vi "Set Voltage and Current.vi"(0 "reference in":refnum<class "Power Supply.lvclass">, 3 "Set Voltage (V)":dbl=5.0, 4 "Set Current (A)":dbl=1.0, 5 "error in (no error)":errorcluster) -> (14 "reference out":refnum<class "Power Supply.lvclass">, 19 "error out":errorcluster)   [LabVIEW 2017, in "Power Supply.lvclass"]
uses:
  Power Supply.lvclass
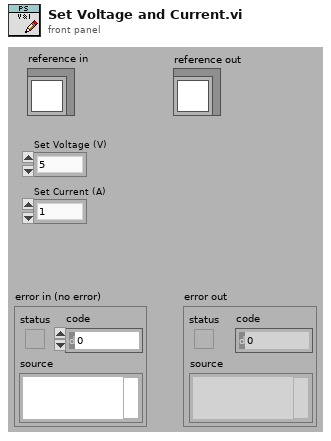
[diagram p1: front panel]
types:
  T1 = typedef "Power Supply.lvclass/ObjectAttributes.ctl" = cluster{"Power Supply Chain VISA Session":refnum<visa-resource-name>, "Power Supply Chain Address":i16, "Power Supply Open/Close Status":bool, "Power Supply Voltage Setting":dbl, "Power Supply Current Setting":dbl, "Power Supply Voltage Reading":dbl, "Power Supply Current Reading":dbl, "Power Supply Status":T2, "Power Supply Error":T3, "Fault Register":u8, "Power Supply Error":bool}
  T2 = typedef "Power Supply.lvclass/Power Supply Status.ctl" = enum16{"Closed", "Open"}
  T3 = typedef "Power Supply.lvclass/Power Supply Error.ctl" = enum16{"None", "Read Error"}
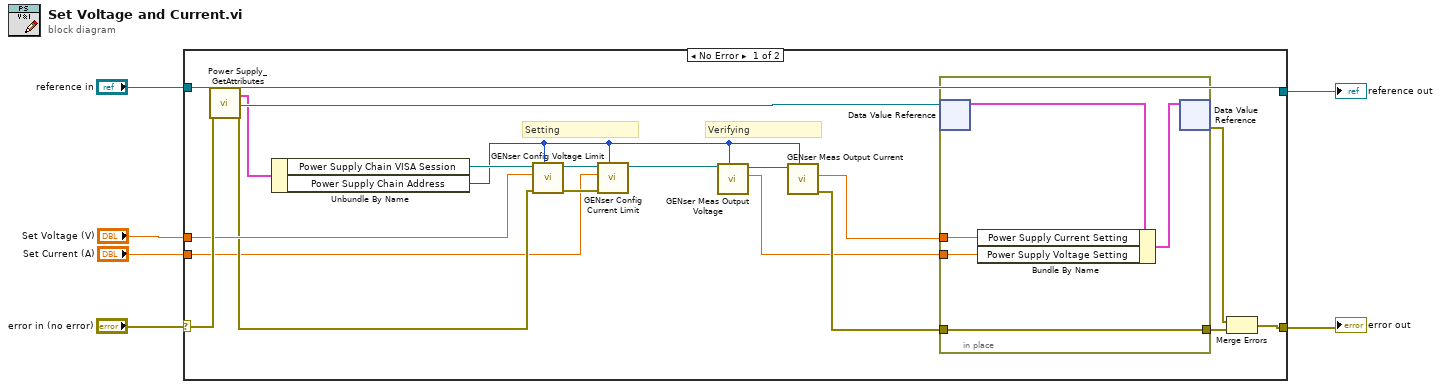
[diagram p0: block diagram]
diagram:
  n1 = case shown="No Error" "error in (no error)" {
    selector: "error in (no error)" -> [w25 w33]
    tunnel: [w22 w33] -> w5
    tunnel: [w23 w32] -> w3
    tunnel: "reference in" -> [w26 w32]
    tunnel: "Set Voltage (V)" -> [w16 _]
    tunnel: "Set Current (A)" -> [w13 _]
    frame No Error {
      # "Verifying"
      # "Setting"
      n2 = call "Power Supply_GetAttributes.vi"("reference in"=w26, "error in (no error)"=w25) -> ("reference out"=w23:refnum<class "Power Supply.lvclass">, "Data"=w20:T1, "DataRef"=w21:refnum<data-value>, "error out"=w15:errorcluster)  [unwired: 14 in]
      n3 = Unbundle By Name(w20) -> ("Power Supply Chain VISA Session"=w17:refnum<visa-resource-name>, "Power Supply Chain Address"=w9:i16)
      n4 = call <instrlib>:"GENser Config Voltage Limit.vi"("GEN Addr"=w9, "error"=w15, "Volt Limit"=w16, "VISA"=w17) -> ("error out"=w19:errorcluster, "VISA out"=w18:refnum<visa-resource-name>)  [unwired: 6 in]
      n5 = call <instrlib>:"GENser Config Current Limit.vi"("GEN Addr"=w9, "error"=w19, "Current Limit"=w13, "VISA"=w18) -> ("VISA out"=w11:refnum<visa-resource-name>)  [unwired: 6 in, 1 out]
      n6 = call <instrlib>:"GENser Meas Output Voltage.vi"("GEN Addr"=w9, "VISA"=w11) -> ("Output Voltage"=w7:dbl, "VISA out"=w10:refnum<visa-resource-name>)  [unwired: 7 in, 1 out]
      n7 = call <instrlib>:"GENser Meas Output Current.vi"("GEN Addr"=w9, "VISA"=w10) -> ("error out"=w12:errorcluster, "Output Current"=w8:dbl)  [unwired: 7 in, 1 out]
      n8 = in-place {
        in-place-border: w8 -> [w29]
        in-place-border: [w28] -> w14
        in-place-border: w12 -> [w28]
        in-place-border: w7 -> [w27]
        n9 = in-place-dvr #1(w21) -> (w31:T1)  [unwired: 1 out]
        n10 = Bundle By Name(cluster=w31, "Power Supply Current Setting"=w29, "Power Supply Voltage Setting"=w27) -> (w30:T1)
        n11 = in-place-dvr #1(w30) -> (w24:errorcluster)  [unwired: 1 out]
      }
      n12 = Merge Errors(w24, w14) -> (w22:errorcluster)
    }
    frame Error {
    }
  }
  "error out" <- w5
  "reference out" <- w3
